vi "cw_4_8.vi"() -> ()   [LabVIEW 2022 SP3]
uses:
  ce2265d8-9254-41ab-a716-7a0b6521e13f.vi
  58160506-7538-4061-b91f-2360cdd73cd9.vi
  <vilib>/Comparison/Less/Less Functor/Less Functor.lvclass
panel:
  out "sorted array":i32[](array[numeric])
  in  "input pages to print":string
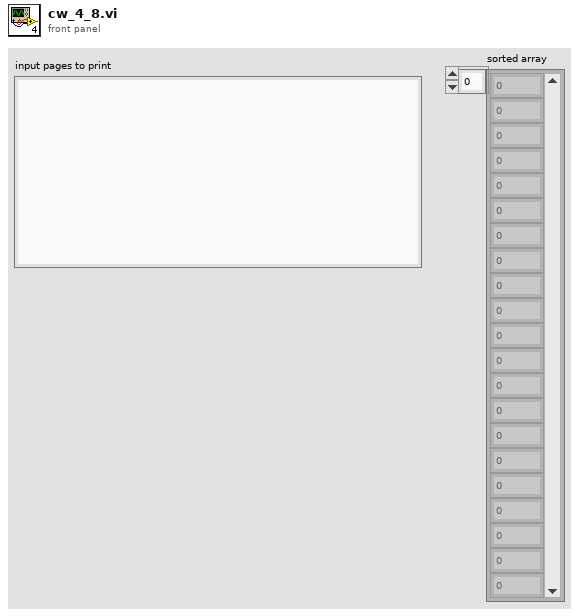
[diagram p1: front panel]
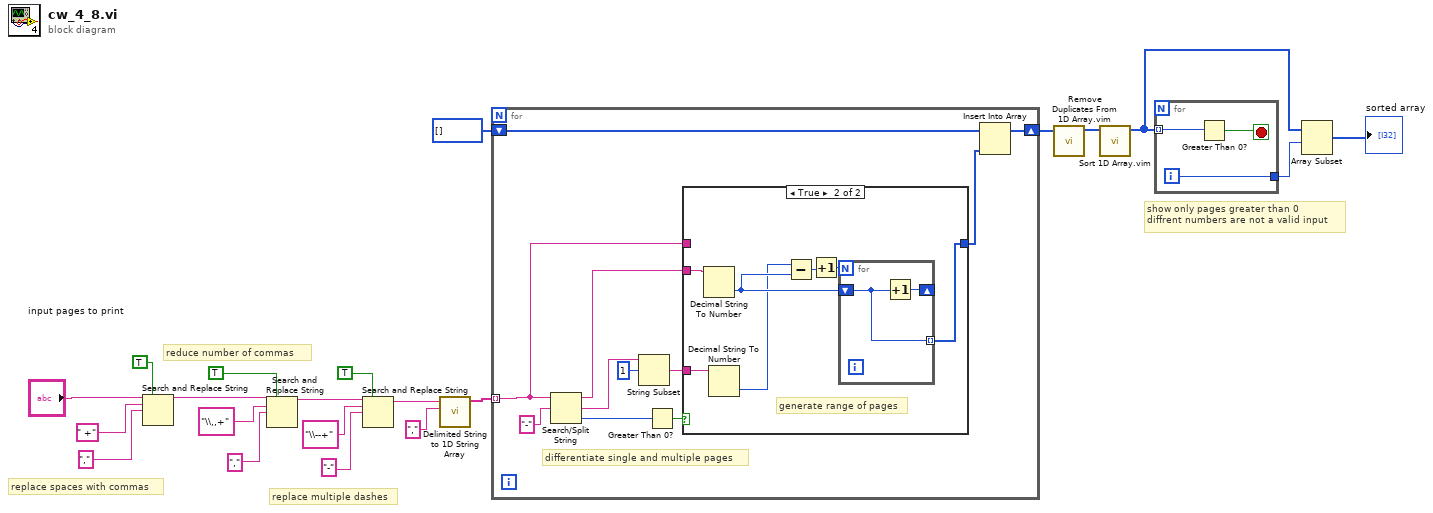
[diagram p0: block diagram]
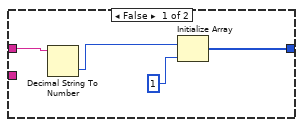
[diagram p2: hidden frame]
diagram:
  # "show only pages greater than 0\ndiffrent numbers are not a valid input"
  # "replace multiple dashes"
  # "reduce number of commas"
  # "replace spaces with commas"
  n1 = Search and Replace String(replace all?=TRUE ("replace all? (F)"), input string="input pages to print", search string=" +", replace string="," ("replace string (\"\")")) -> (result string=w16:string)  [unwired: 4 in, 3 out]
  n2 = Search and Replace String(replace all?=TRUE ("replace all? (F)"), input string=w16, search string="\\,,+", replace string="," ("replace string (\"\")")) -> (result string=w8:string)  [unwired: 4 in, 3 out]
  n3 = Search and Replace String(replace all?=TRUE ("replace all? (F)"), input string=w8, search string="\\--+", replace string="-" ("replace string (\"\")")) -> (result string=w7:string)  [unwired: 4 in, 3 out]
  n4 = call <vilib>:"Delimited String to 1D String Array.vi"("delimiter"=",", "delimited string"=w7) -> ("string array"=w20:string[])  [unwired: 9 in]
  n5 = for {
    tunnel: w20 -> [w26] mode=indexing
    shift-right: [w31] -> w6
    shift-left: i32[] [] -> [w32]
    # "differentiate single and multiple pages"
    n6 = Search/Split String(string=w26, search string/char (-)="-") -> (substring before match=w27:string, match + rest of string=w24:string, offset of match=w29:i32)  [unwired: 1 in]
    n7 = String Subset(string=w24, offset (0)=1) -> (substring=w22:string)  [unwired: 1 in]
    n8 = Greater Than 0?(x=w29) -> (x > 0?=w28:bool)
    n9 = case shown="True" w28 {
      tunnel: w27 -> [_ w43]
      tunnel: w26 -> [w35 _]
      tunnel: [w34 w39] -> w25
      tunnel: w22 -> [_ w42]
      frame False {
        n10 = Decimal String To Number(string=w35) -> (number=w33:i32)  [unwired: 2 in, 1 out]
        n11 = Initialize Array(w33, 1 ("dimension size")) -> (w34:i32[])
      }
      frame True {
        # "generate range of pages"
        n12 = Decimal String To Number(string=w43) -> (number=w38:i32)  [unwired: 2 in, 1 out]
        n13 = Decimal String To Number(string=w42) -> (number=w37:i32)  [unwired: 2 in, 1 out]
        n14 = Subtract(x=w37, y=w38) -> (x-y=w41:i32)
        n15 = Increment(x=w41) -> (x+1=w40:i32)
        n16 = for {
          N: w40 -> [_]
          shift-right: [w45] -> _
          shift-left: w38 -> [w44]
          tunnel: [w44] -> w39 mode=indexing
          n17 = Increment(x=w44) -> (x+1=w45:i32)
        }
      }
    }
    n18 = Insert Into Array(array=w32, new element=w25) -> (w31:i32[])  [unwired: 1 in]
  }
  n19 = call "Remove Duplicates From 1D Array.vim"("array"=w6) -> ("array with duplicates removed"=w5:i32[])  [unwired: 10 in]
  n20 = call "Sort 1D Array.vim"("unsorted array"=w5) -> ("sorted array"=w3:i32[])  [unwired: 10 in]
  n21 = for {
    tunnel: w3 -> [w48] mode=indexing
    tunnel: [w46] -> w2
    i -> [w46]
    stop <- w47 stop-if-true
    n22 = Greater Than 0?(x=w48) -> (x > 0?=w47:bool)
  }
  n23 = Array Subset(array=w3, index=w2) -> (→"sorted array":i32[])  [unwired: 1 in]
